vi "user output.vi"(7 "FPGA Interface":T1, 8 "error in":errorcluster, 11 "Outputs to system":T2) -> (0 "error out":errorcluster)   [LabVIEW 2015, in "GPIC ScaleAndLimit runtime.lvclass"]
uses:
  GPIC ScaleAndLimit runtime.lvclass
  output user data.ctl
  Interface/FPGAInterface.ctl
  <vilib>/Utility/error.llb/Error Cluster From Error Code.vi
  <vilib>/rvi/errors/niLvFpgaAdjustHostInterfaceError.vi
  <vilib>/rvi/interface/nirviReadWriteControl/nirviReadWriteControl.xnode
  Interface/ScaleAndLimitInterface.lvlib
  NiFpgaLv.dll
  <vilib>/rvi/interface/Simulation/niFpgaSimulationCallBeginRW.vi
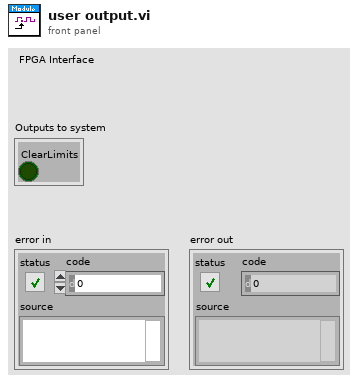
[diagram p1: front panel]
types:
  T1 = typedef "ScaleAndLimitInterface.lvlib/FPGAInterface.ctl" = refnum<k20>
  T2 = typedef "GPIC ScaleAndLimit runtime.lvclass/output user data.ctl" = cluster{"ClearLimits":bool}
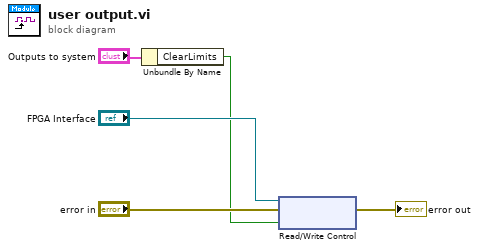
[diagram p0: block diagram]
diagram:
  n1 = Unbundle By Name("Outputs to system") -> ("ClearLimits"=w2:bool)
  n2 = xnode "Read/Write Control"("FPGA VI Reference In"="FPGA Interface", "error in"="error in", "ClearLimits"=w2) -> ("error out"=→"error out":errorcluster)  [unwired: 1 out]
